vi "ATS9350_NPT.vi"() -> ()   [LabVIEW 2018]
panel:
  out "error out":errorcluster
  out "Graph":u16[](graph)
  in  "stop":bool
  # "Connect proper signal to channel A before starting acquisition\n(e.g. 1Vpp 1kHz sine wave)"
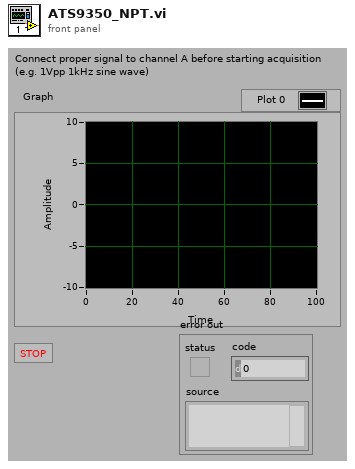
[diagram p1: front panel]
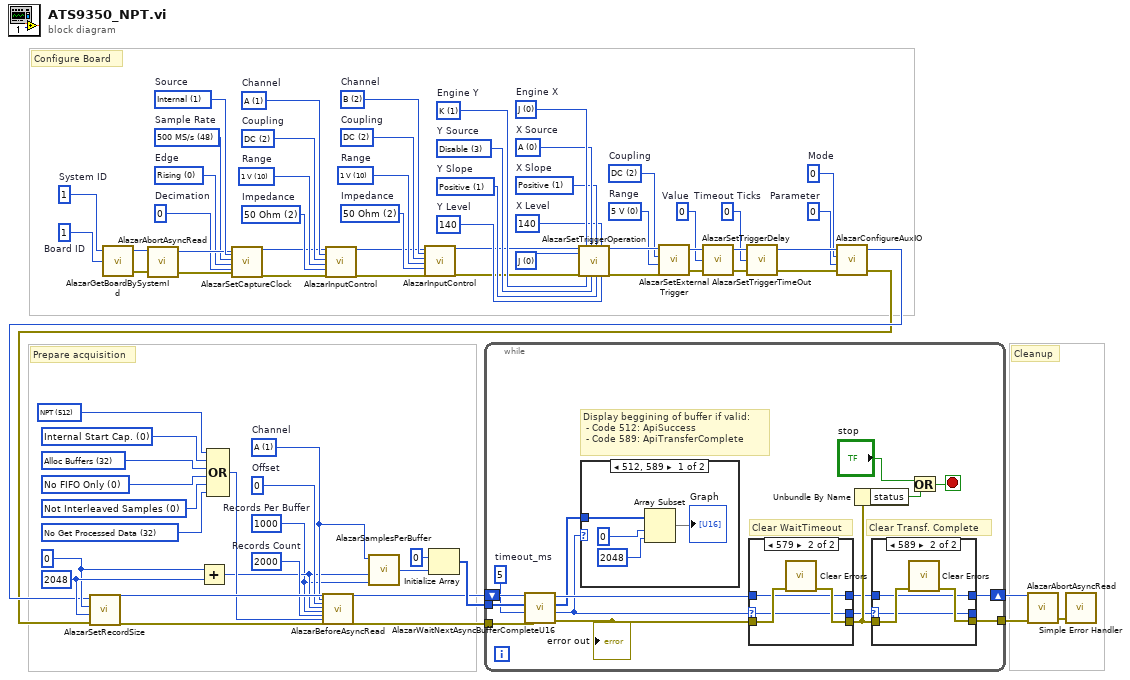
[diagram p0: block diagram]
diagram:
  w35 = u32 2 items=["50 Ohm"=2]  # Impedance
  w34 = u32 10 items=["40 mV"=2, "100 mV"=5, "200 mV"=6, "400 mV"=7, "1 V"=10, "2 V"=11, "4 V"=12]  # Range
  w36 = u32 2 items=["AC"=1, "DC"=2]  # Coupling
  w37 = u8 2 items=["A"=1, "B"=2, "C"=4, "D"=8]  # Channel
  w13 = u32 0  # Parameter
  w12 = u32 0  # Mode
  w11 = u32 0  # Timeout Ticks
  w18 = u32 0  # Value
  w22 = u32 0 items=["5 V", "1 V", "TTL"]  # Range
  w21 = u32 2 items=["AC"=1, "DC"=2]  # Coupling
  w25 = u32 140  # Y Level
  w26 = u32 1 items=["Positive"=1, "Negative"=2]  # Y Slope
  w27 = u32 3 items=["A", "B", "External", "Disable", "C", "D"]  # Y Source
  w29 = u32 140  # X Level
  w30 = u32 1 items=["Positive"=1, "Negative"=2]  # X Slope
  w31 = u32 0 items=["A", "B", "External", "Disable", "C", "D"]  # X Source
  w28 = u32 1 items=["J", "K"]  # Engine Y
  w32 = u32 0 items=["J", "K"]  # Engine X
  w33 = u32 0 items=["J", "K", "J OR K", "J AND K", "J XOR K", "J AND NOT K", "NOT J AND K"] ("Op.")
  w40 = u32 2 items=["50 Ohm"=2]  # Impedance
  w41 = u32 10 items=["40 mV"=2, "100 mV"=5, "200 mV"=6, "400 mV"=7, "1 V"=10, "2 V"=11, "4 V"=12]  # Range
  w42 = u32 2 items=["AC"=1, "DC"=2]  # Coupling
  w43 = u8 1 items=["A"=1, "B"=2, "C"=4, "D"=8]  # Channel
  w45 = u32 0  # Decimation
  w46 = u32 0 items=["Rising", "Falling"]  # Edge
  w47 = u32 48 items=["1 kS/s"=1, "2 kS/s"=2, "5 kS/s"=4, "10 kS/s"=8, "20 kS/s"=10, "50 kS/s"=12, "100 kS/s"=14, "200 kS/s"=16, "500 kS/s"=18, "1 MS/s"=20, "2 MS/s"=24, "5 MS/s"=26, "10 MS/s"=28, "20 MS/s"=30, "50 MS/s"=34, "100 MS/s"=36, "125 MS/s"=37, "250 MS/s"=43, "500 MS/s"=48, "USER_DEF"=0]  # Sample Rate
  w49 = u32 1 items=["Internal"=1, "Fast External"=2, "Medium External"=3, "Slow External"=4, "External AC"=5, "External DC"=6, "External 10MHz"=7]  # Source
  w53 = u32 1  # Board ID
  w52 = u32 1  # System ID
  w61 = u32 2000  # Records Count
  w1 = u32 1000  # Records Per Buffer
  w62 = u32 0  # Offset
  w3 = u32 1 items=["A"=1, "B"=2, "A + B"=3, "C"=4, "A + C"=5, "A + B"=6, "D"=8, "A + D"=9, "B + D"=10, "C + D"=12, "A + B + C + D"=15]  # Channel
  w67 = u32 2048 ("Post-trigger Samples")
  w66 = u32 0 ("Pre-trigger Samples")
  w73 = u32 32 items=["No Get Processed Data"=32, "Get Processed Data"=8192]
  w72 = u32 0 items=["Not Interleaved Samples"=0, "Interleave Samples"=4096]
  w68 = u32 0 items=["No FIFO Only"=0, "FIFO Only"=2048]
  w71 = u32 32 items=["Alloc Buffers"=32]
  w70 = u32 0 items=["Internal Start Cap.", "External Start Cap."]
  w69 = u32 512 items=["Traditional"=0, "NPT"=512, "Continuous"=256, "Triggered Streaming"=1024]
  # "Configure Board"
  # "Cleanup"
  # "Prepare acquisition"
  n1 = call "AlazarGetBoardBySystemId.vi"("Board ID"=w53, "System ID"=w52) -> ("error out"=w50:errorcluster, "Handle"=w51:u32)  [unwired: 1 in, 1 out]
  n2 = call "AlazarAbortAsyncRead.vi"("Handle"=w51, "error in (no error)"=w50) -> ("Handle"=w48:u32, "error out"=w44:errorcluster)  [unwired: 1 out]
  n3 = Add(x=w66, y=w67) -> (x+y=w2:u32)
  n4 = Compound Arithmetic op=OR(w69, w70, w71, w68, w72, w73) -> (w63:u32)
  n5 = call "AlazarSetCaptureClock.vi"("Handle"=w48, "Source"=w49, "Sample Rate"=w47, "Edge"=w46, "Decimation"=w45, "error in (no error)"=w44) -> ("Handle"=w39:u32, "error out"=w38:errorcluster)  [unwired: 11 in, 1 out]
  n6 = call "AlazarInputControl.vi"("Handle"=w39, "Channel"=w43, "Coupling"=w42, "Range"=w41, "Impedance"=w40, "error in (no error)"=w38) -> ("Handle"=w10:u32, "error out"=w9:errorcluster)  [unwired: 11 in, 1 out]
  n7 = call "AlazarSamplesPerBuffer.vi"("Records Per Buffer"=w1, "Samples Per Record"=w2, "Channel Mask"=w3) -> ("Samples Per Buffer"=w4:u32)  [unwired: 1 in]
  n8 = call "AlazarInputControl.vi"("Handle"=w10, "Channel"=w37, "Coupling"=w36, "Range"=w34, "Impedance"=w35, "error in (no error)"=w9) -> ("Handle"=w7:u32, "error out"=w8:errorcluster)  [unwired: 11 in, 1 out]
  n9 = Initialize Array(u16 0, w4) -> (w59:u16[])
  n10 = call "AlazarSetTriggerOperation.vi"("Handle"=w7, "Trigger Operation"=w33, "error in (no error)"=w8, "Trigger Engine 1"=w32, "Trigger Engine 2"=w28, "Source 1"=w31, "Source 2"=w27, "Slope 1"=w30, "Slope 2"=w26, "Level 1"=w29, "Level 2"=w25) -> ("Handle"=w24:u32, "error out"=w23:errorcluster)  [unwired: 6 in, 1 out]
  n11 = call "AlazarSetExternalTrigger.vi"("error in (no error)"=w23, "Range ID"=w22, "Coupling ID"=w21, "Handle"=w24) -> ("error out"=w19:errorcluster, "Handle"=w20:u32)  [unwired: 1 out]
  n12 = call "AlazarSetTriggerDelay.vi"("error in (no error)"=w19, "Delay"=w18, "Handle"=w20) -> ("error out"=w16:errorcluster, "Handle"=w17:u32)  [unwired: 1 out]
  n13 = call "AlazarSetTriggerTimeOut.vi"("error in (no error)"=w16, "Timeout Ticks"=w11, "Handle"=w17) -> ("error out"=w14:errorcluster, "Handle"=w15:u32)  [unwired: 1 out]
  n14 = call "AlazarConfigureAuxIO.vi"("error in (no error)"=w14, "Parameter"=w13, "Mode"=w12, "Handle"=w15) -> ("error out"=w5:errorcluster, "Handle"=w6:u32)  [unwired: 1 out]
  n15 = call "AlazarSetRecordSize.vi"("error in (no error)"=w5, "Post-trigger Samples"=w67, "Pre-trigger Samples"=w66, "Handle"=w6) -> ("error out"=w64:errorcluster, "Handle"=w65:u32)  [unwired: 1 out]
  n16 = call "AlazarBeforeAsyncRead.vi"("Handle"=w65, "Channel Select"=w3, "Transfer Offset"=w62, "Transfer Length"=w2, "Records Per Buffer"=w1, "Records Per Acquisition"=w61, "Flags"=w63, "error in (no error)"=w64) -> ("Handle"=w58:u32, "error out"=w57:errorcluster)  [unwired: 17 in, 1 out]
  n17 = while {
    tunnel: w59 -> [w89]
    tunnel: w57 -> [w86]
    tunnel: [w78] -> w54
    shift-right: [w79] -> w55
    shift-left: w58 -> [w88]
    stop <- w82 stop-if-true
    w87 = u32 5  # timeout_ms
    # "Display beggining of buffer if valid:\n - Code 512: ApiSuccess\n - Code 589: ApiTransferComplete"
    # "Clear Transf. Complete"
    # "Clear WaitTimeout"
    n18 = call "AlazarWaitNextAsyncBufferCompleteU16.vi"("error in (no error)"=w86, "Timeout (ms)"=w87, "Buffer"=w89, "Handle"=w88) -> ("error out"=w75:errorcluster, "Return Code"=w74:u32, "Buffer"=w76:u16[], "Handle"=w77:u32)
    "error out" <- w75
    n19 = case shown="512, 589" w74 {
      tunnel: w76 -> [w90 _]
      frame 512, 589 {
        n20 = Array Subset(array=w90, index=0, length=2048) -> (→"Graph":u16[])
      }
      frame Default {
      }
    }
    n21 = case shown="579" w74 {
      selector: w74 -> [w102 w104]
      tunnel: w75 -> [w101 w107]
      tunnel: [w101 w106] -> w85
      tunnel: [w103 w105] -> w84
      tunnel: w77 -> [w103 w105]
      tunnel: [w102 w104] -> w83
      frame 0, Default {
      }
      frame 579 {
        n22 = call <vilib>:"Clear Errors.vi"("error in (no error)"=w107) -> ("error out"=w106:errorcluster)  [unwired: 5 in, 1 out]
      }
    }
    n23 = Unbundle By Name(w85) -> ("status"=w80:bool)
    n24 = case shown="589" w83 {
      selector: w83 -> [w95 w97]
      tunnel: w85 -> [w94 w100]
      tunnel: [w94 w99] -> w78
      tunnel: [w96 w98] -> w79
      tunnel: w84 -> [w96 w98]
      tunnel: [w95 w97] -> _
      frame 0, Default {
      }
      frame 589 {
        n25 = call <vilib>:"Clear Errors.vi"("error in (no error)"=w100) -> ("error out"=w99:errorcluster)  [unwired: 5 in, 1 out]
      }
    }
    n26 = Or(x="stop", y=w80) -> (x .or. y?=w82:bool)
  }
  n27 = call "AlazarAbortAsyncRead.vi"("Handle"=w55, "error in (no error)"=w54) -> ("error out"=w56:errorcluster)  [unwired: 2 out]
  n28 = call <vilib>:"Simple Error Handler.vi"("error in (no error)"=w56) -> ()  [unwired: 4 in, 5 out]
